vi "ProcessRun.vi"(5 "EndTime":timestamp, 7 "StartTime":timestamp, 8 "error in":errorcluster, 11 "ProcessRun":refnum<class "ProcessRun.lvclass">) -> (0 "error out":errorcluster, 3 "Passed":bool)   [LabVIEW 2020]
uses:
  <vilib>/Averna/ProligentResultProcessor/ProligentResultProcessor.lvlibp/ProcessRun/ProcessRun.lvclass
  <vilib>/Averna/ProligentResultProcessor/ProligentResultProcessor.lvlibp/ProcessRun/SetProcessRunId.vi
  <vilib>/Averna/ProligentResultProcessor/ProligentResultProcessor.lvlibp/ProcessRun/SetProcessFullName.vi
  <vilib>/Averna/ProligentResultProcessor/ProligentResultProcessor.lvlibp/ProcessRun/SetProcessVersion.vi
  <vilib>/Averna/ProligentResultProcessor/ProligentResultProcessor.lvlibp/ProcessRun/SetProductUnitIdentifier.vi
  <vilib>/Averna/ProligentResultProcessor/ProligentResultProcessor.lvlibp/ProcessRun/SetProductFullName.vi
  <vilib>/Averna/ProligentResultProcessor/ProligentResultProcessor.lvlibp/ProcessRun/SetProcessRunStatus.vi
  <vilib>/Averna/ProligentResultProcessor/ProligentResultProcessor.lvlibp/ProcessRun/SetProcessRunStartTime.vi
  <vilib>/Averna/ProligentResultProcessor/ProligentResultProcessor.lvlibp/ProcessRun/SetProcessRunEndTime.vi
  <vilib>/Averna/ProligentResultProcessor/ProligentResultProcessor.lvlibp/ProcessRun/SetProcessMode.vi
  <vilib>/Averna/ProligentResultProcessor/ProligentResultProcessor.lvlibp/ProcessRun/GetProcessRunId.vi
  <vilib>/Averna/ProligentResultProcessor/ProligentResultProcessor.lvlibp/ProcessRun/GetProcessFullName.vi
  <vilib>/Averna/ProligentResultProcessor/ProligentResultProcessor.lvlibp/ProcessRun/GetProcessVersion.vi
  <vilib>/Averna/ProligentResultProcessor/ProligentResultProcessor.lvlibp/ProcessRun/GetProductUnitIdentifier.vi
  <vilib>/Averna/ProligentResultProcessor/ProligentResultProcessor.lvlibp/ProcessRun/GetProductFullName.vi
  <vilib>/Averna/ProligentResultProcessor/ProligentResultProcessor.lvlibp/ProcessRun/GetProcessRunStatus.vi
  <vilib>/Averna/ProligentResultProcessor/ProligentResultProcessor.lvlibp/ProcessRun/GetProcessRunStartTime.vi
  <vilib>/Averna/ProligentResultProcessor/ProligentResultProcessor.lvlibp/ProcessRun/GetProcessRunEndTime.vi
  <vilib>/Averna/ProligentResultProcessor/ProligentResultProcessor.lvlibp/ProcessRun/GetProcessMode.vi
  <vilib>/Averna/ProligentResultProcessor/ProligentResultProcessor.lvlibp/ProcessRun/GetOperationRuns.vi
  <vilib>/Averna/ProligentResultProcessor/ProligentResultProcessor.lvlibp/ProcessRun/GetOperationCycles.vi
  <vilib>/Averna/ProligentResultProcessor/ProligentResultProcessor.lvlibp/ProcessRun/GetFailureReferences.vi
  <vilib>/Averna/ProligentResultProcessor/ProligentResultProcessor.lvlibp/ProcessRun/GetCustomData.vi
  <vilib>/Averna/ProligentResultProcessor/ProligentResultProcessor.lvlibp/OperationRun/OperationRun.lvclass
  <vilib>/Averna/ProligentResultProcessor/ProligentResultProcessor.lvlibp/OperationCycle/OperationCycle.lvclass
  <vilib>/Averna/ProligentResultProcessor/ProligentResultProcessor.lvlibp/Failure/FailureReference/FailureReference.lvclass
  <vilib>/Averna/ProligentResultProcessor/ProligentResultProcessor.lvlibp/Model/CustomData/CustomData.lvclass
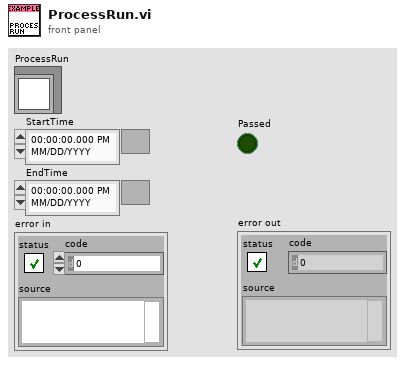
[diagram p1: front panel]
types:
  T1 = enum16{"PASS", "FAIL", "NOT_COMPLETED", "ABORTED"}
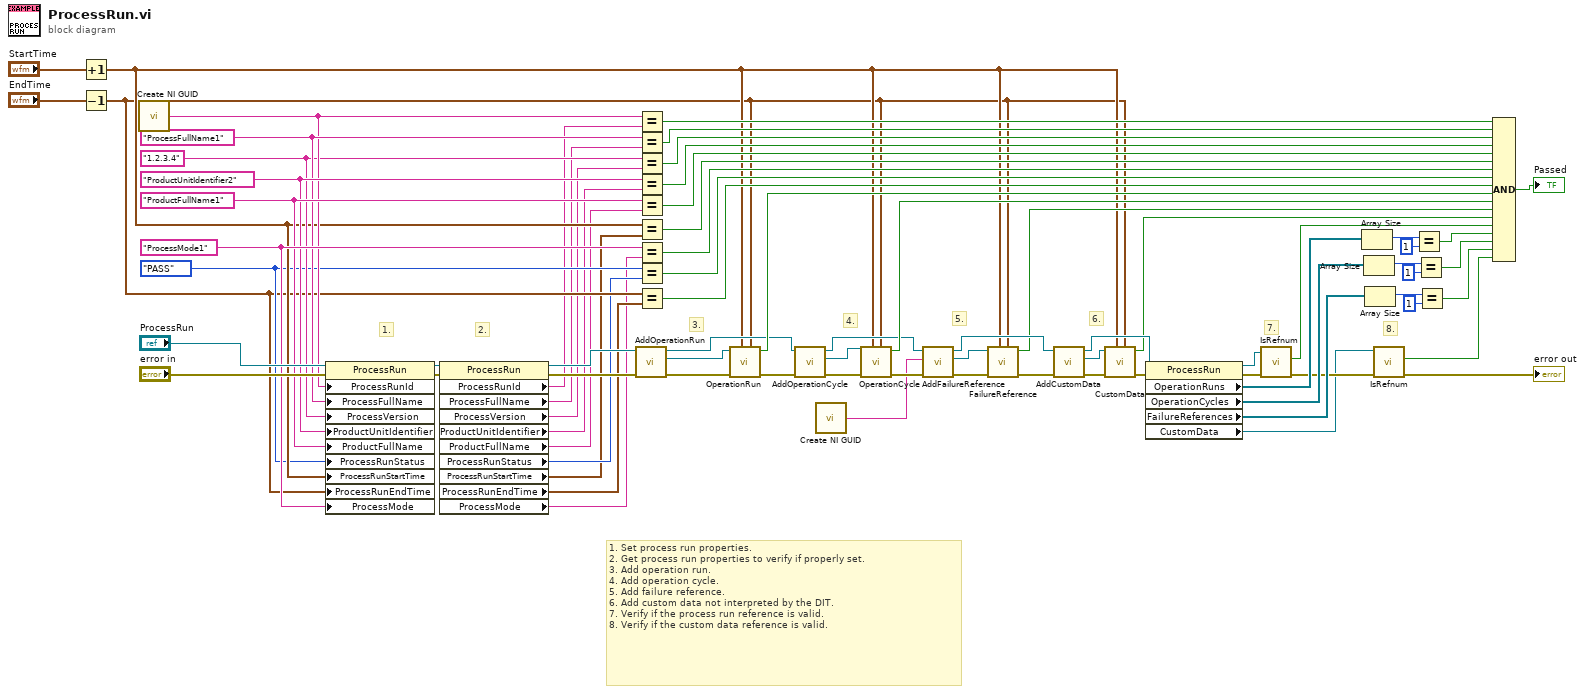
[diagram p0: block diagram]
diagram:
  w47 = "1.2.3.4"
  w28 = T1."PASS" ("ProcessRunStatus")
  w74 = "ProcessMode1"
  w73 = "ProductFullName1"
  w72 = "ProductUnitIdentifier2"
  w71 = "ProcessFullName1"
  # "8."
  # "7."
  # "6."
  # "5."
  # "4."
  # "3."
  # "1. Set process run properties.\n2. Get process run properties to verify if properly set.\n3. Add operation run.\n4. Add operation cycle.\n5. Add failure reference.\n6. Add custom data not interpreted by the DIT.\n7. Verify if the process run reference is valid.\n8. Verify if the custom data reference is valid."
  # "2."
  # "1."
  n1 = Increment(x="StartTime") -> (x+1=w30:timestamp)
  n2 = Decrement(x="EndTime") -> (x-1=w27:timestamp)
  n3 = call <vilib>:"Create NI GUID.vi"() -> ("NI GUID"=w49:string)
  n4 = property class="ProcessRun"(reference="ProcessRun", error in="error in", "ProcessRunId"=w49, "ProcessFullName"=w71, "ProcessVersion"=w47, "ProductUnitIdentifier"=w72, "ProductFullName"=w73, "ProcessRunStatus"=w28, "ProcessRunStartTime"=w30, "ProcessRunEndTime"=w27, "ProcessMode"=w74) -> (reference out=w26:refnum<class "ProcessRun.lvclass">, error out=w25:errorcluster)
  n5 = property class="ProcessRun"(reference=w26, error in=w25) -> (reference out=w23:refnum<class "ProcessRun.lvclass">, error out=w24:errorcluster, "ProcessRunId"=w22:string, "ProcessFullName"=w21:string, "ProcessVersion"=w20:string, "ProductUnitIdentifier"=w19:string, "ProductFullName"=w18:string, "ProcessRunStatus"=w17:T1, "ProcessRunStartTime"=w16:timestamp, "ProcessRunEndTime"=w15:timestamp, "ProcessMode"=w14:string)
  n6 = call <vilib>:"AddOperationRun.vi"("error in"=w24, "ProcessRun in"=w23) -> ("error out"=w56:errorcluster, "OperationRun"=w57:refnum<class "OperationRun.lvclass">, "ProcessRun out"=w41:refnum<class "ProcessRun.lvclass">)  [unwired: 7 in]
  n7 = Equal?(x=w49, y=w22) -> (x = y?=w50:bool)
  n8 = Equal?(x=w71, y=w21) -> (x = y?=w66:bool)
  n9 = Equal?(x=w47, y=w20) -> (x = y?=w48:bool)
  n10 = Equal?(x=w72, y=w19) -> (x = y?=w65:bool)
  n11 = Equal?(x=w73, y=w18) -> (x = y?=w64:bool)
  n12 = Equal?(x=w30, y=w16) -> (x = y?=w63:bool)
  n13 = Equal?(x=w74, y=w14) -> (x = y?=w62:bool)
  n14 = Equal?(x=w28, y=w17) -> (x = y?=w61:bool)
  n15 = Equal?(x=w27, y=w15) -> (x = y?=w60:bool)
  n16 = call "OperationRun.vi"("EndTime"=w27, "StartTime"=w30, "error in"=w56, "OperationRun"=w57) -> ("error out"=w42:errorcluster, "Passed"=w55:bool)  [unwired: 6 in]
  n17 = call <vilib>:"AddOperationCycle.vi"("error in"=w42, "ProcessRun in"=w41) -> ("error out"=w40:errorcluster, "OperationRun"=w39:refnum<class "OperationCycle.lvclass">, "ProcessRun out"=w36:refnum<class "ProcessRun.lvclass">)  [unwired: 7 in]
  n18 = call <vilib>:"Create NI GUID.vi"() -> ("NI GUID"=w29:string)
  n19 = call "OperationCycle.vi"("EndTime"=w27, "StartTime"=w30, "error in"=w40, "OperationRun"=w39) -> ("error out"=w37:errorcluster, "Passed"=w38:bool)  [unwired: 6 in]
  n20 = call <vilib>:"AddFailureReference.vi"("error in"=w37, "Id"=w29, "ProcessRun in"=w36) -> ("error out"=w34:errorcluster, "OperationRun"=w32:refnum<class "FailureReference.lvclass">, "ProcessRun out"=w35:refnum<class "ProcessRun.lvclass">)  [unwired: 6 in]
  n21 = call "FailureReference.vi"("EndTime"=w27, "StartTime"=w30, "error in"=w34, "FailureReference"=w32) -> ("error out"=w33:errorcluster, "Passed"=w31:bool)  [unwired: 6 in]
  n22 = call <vilib>:"AddCustomData.vi"("error in"=w33, "Defect in"=w35) -> ("error out"=w46:errorcluster, "CustomData"=w45:refnum<class "CustomData.lvclass">, "Defect out"=w44:refnum<class "ProcessRun.lvclass">)  [unwired: 7 in]
  n23 = call "CustomData.vi"("EndTime"=w27, "StartTime"=w30, "error in"=w46, "CustomData"=w45) -> ("error out"=w43:errorcluster, "Passed"=w1:bool)  [unwired: 6 in]
  n24 = property class="ProcessRun"(reference=w44, error in=w43) -> (reference out=w52:refnum<class "ProcessRun.lvclass">, error out=w67:errorcluster, "OperationRuns"=w68:refnum<class "OperationRun.lvclass">[], "OperationCycles"=w9:refnum<class "OperationCycle.lvclass">[], "FailureReferences"=w8:refnum<class "FailureReference.lvclass">[], "CustomData"=w3:refnum<class "CustomData.lvclass">)
  n25 = call <vilib>:"IsRefnum.vi"("error in"=w67, "ProcessRun in"=w52) -> ("error out"=w5:errorcluster, "IsRefnum"=w51:bool)  [unwired: 7 in, 1 out]
  n26 = Array Size(array=w68) -> (size(s)=w70:i32)
  n27 = Array Size(array=w9) -> (size(s)=w12:i32)
  n28 = Array Size(array=w8) -> (size(s)=w11:i32)
  n29 = call <vilib>:"IsRefnum.vi"("error in"=w5, "CustomDataType in"=w3) -> ("error out"=→"error out":errorcluster, "IsRefnum"=w2:bool)  [unwired: 7 in, 1 out]
  n30 = Equal?(x=w70, y=1) -> (x = y?=w59:bool)
  n31 = Equal?(x=w12, y=1) -> (x = y?=w7:bool)
  n32 = Equal?(x=w11, y=1) -> (x = y?=w6:bool)
  n33 = Compound Arithmetic op=AND(w50, w66, w48, w65, w64, w63, w62, w61, w60, w55, w38, w31, w1, w51, w59, w7, w6, w2) -> (→"Passed":bool)
